vi "Grab Image and Find peoplel.vi"(8 "error in (no error)":errorcluster, 11 "ball tracking refs in":T2={"acquired image"=refnum, "threshold image"=refnum, "Video Handle out"=0, "Kinect Handle"=0, "Video and Depth config"={"Video Resolution"=enum."FREENECT_RESOLUTION_LOW", "Video Format"=enum."FREENECT_VIDEO_RGB", "Depth Format"=enum."FREENECT_DEPTH_11BIT", "Depth Resolution"=enum."FREENECT_RESOLUTION_MEDIUM"}}) -> (0 "error out":errorcluster, 1 "ball pixel position":T1, 2 "ball found?":bool, 3 "ball tracking refs out":T2={"acquired image"=refnum, "threshold image"=refnum, "Video Handle out"=0, "Kinect Handle"=0, "Video and Depth config"={"Video Resolution"=enum."FREENECT_RESOLUTION_LOW", "Video Format"=enum."FREENECT_VIDEO_RGB", "Depth Format"=enum."FREENECT_DEPTH_11BIT", "Depth Resolution"=enum."FREENECT_RESOLUTION_MEDIUM"}}, 4 "image resolution":cluster{"x":i32, "y":i32}={"x"=640, "y"=480})   [LabVIEW 2014]
doc: "This VI grabs an image from the camera, then estimates the locatation and distance of a green tennis ball in the image."
uses:
  Ball Tracking Image Refs.ctl
  <vilib>/vision/Image Controls.llb/IMAQ Image.ctl
  KinectProject/subVIs/Video Resolution Control.ctl
  KinectProject/subVIs/Video Format Control.ctl
  KinectProject/subVIs/Depth Format Control.ctl
  KinectProject/subVIs/Depth Resolution Control.ctl
  Ball Pixel Info.ctl
  Ball Tracking Globals.vi
  <vilib>/vision/NI_Vision_Development_Module.lvlib
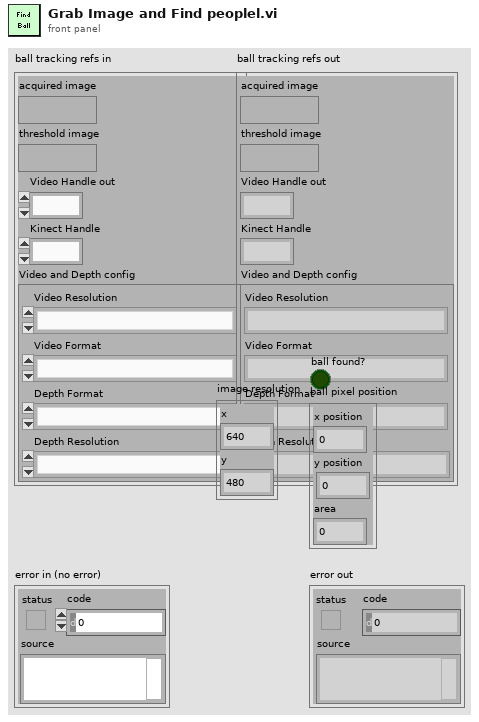
[diagram p1: front panel]
types:
  T1 = typedef "Ball Pixel Info.ctl" = cluster{"x position":dbl, "y position":dbl, "area":dbl}
  T2 = typedef "Ball Tracking Image Refs.ctl" = cluster{"acquired image":T3, "threshold image":T3, "Video Handle out":i64, "Kinect Handle":i64, "Video and Depth config":cluster{"Video Resolution":T4, "Video Format":T5, "Depth Format":T6, "Depth Resolution":T7}}
  T3 = typedef "IMAQ Image.ctl" = refnum<image>
  T4 = typedef "Video Resolution Control.ctl" = enum32{"FREENECT_RESOLUTION_LOW", "FREENECT_RESOLUTION_MEDIUM", "FREENECT_RESOLUTION_HIGH"}
  T5 = typedef "Video Format Control.ctl" = enum32{"FREENECT_VIDEO_RGB", "FREENECT_VIDEO_BAYER", "FREENECT_VIDEO_IR_8BIT", "FREENECT_VIDEO_IR_10BIT", "FREENECT_VIDEO_IR_10BIT_PACKED", "FREENECT_VIDEO_YUV_RGB", "FREENECT_VIDEO_YUV_RAW"}
  T6 = typedef "Depth Format Control.ctl" = enum32{"FREENECT_DEPTH_11BIT", "FREENECT_DEPTH_10BIT", "FREENECT_DEPTH_11BIT_PACKED", "FREENECT_DEPTH_10BIT_PACKED", "FREENECT_DEPTH_REGISTERED", "FREENECT_DEPTH_MM"}
  T7 = typedef "Depth Resolution Control.ctl" = enum16{"FREENECT_RESOLUTION_TINY", "FREENECT_RESOLUTION_LOW", "FREENECT_RESOLUTION_MEDIUM"}
  T8 = typedef "Particle Parameters" = i32
  T9 = cluster{"Video Resolution":T4, "Video Format":T5, "Depth Format":T6, "Depth Resolution":T7}
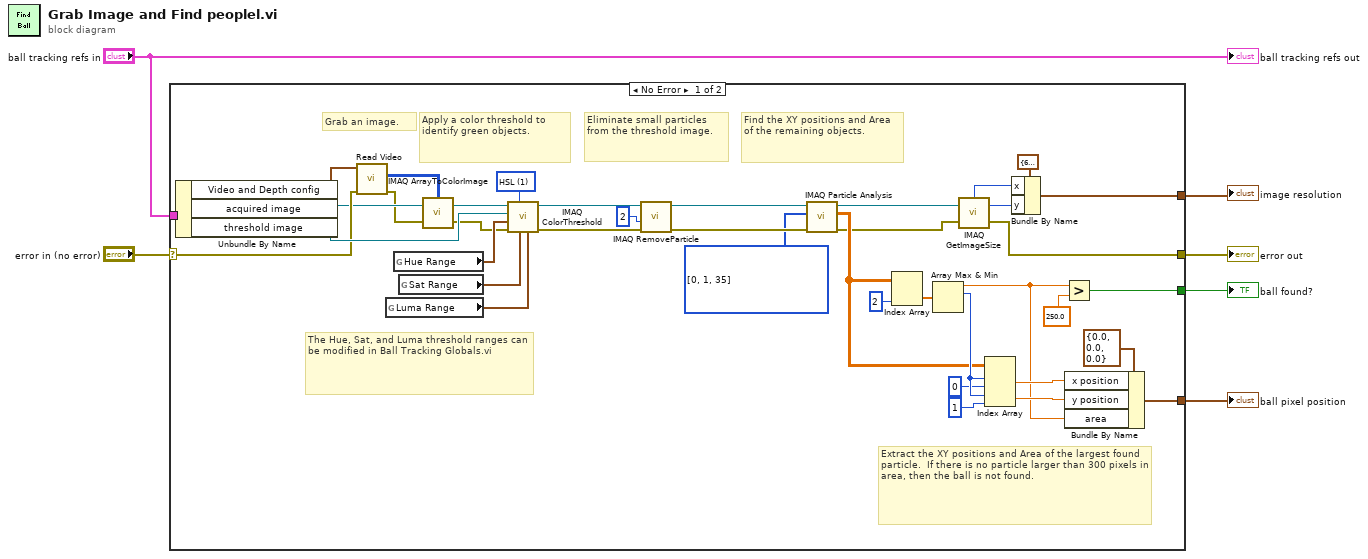
[diagram p0: block diagram]
diagram:
  n1 = case shown="No Error" "error in (no error)" {
    selector: "error in (no error)" -> [w13 w46]
    tunnel: "ball tracking refs in" -> [w45 _]
    tunnel: [w21 w46] -> w5
    tunnel: [w33 _] -> w3
    tunnel: [w25 _] -> w2
    tunnel: [w17 _] -> w1
    frame No Error {
      w37 = T8[] [0, 1, 35] items=["Center of Mass X", "Center of Mass Y", "First Pixel X", "First Pixel Y", "Bounding Rect Left", "Bounding Rect Top", "Bounding Rect Right", "Bounding Rect Bottom", "Max Feret Diameter Start X", "Max Feret Diameter Start Y", "Max Feret Diameter End X", "Max Feret Diameter End Y", "Max Horiz. Segment Length Left", "Max Horiz. Segment Length Right", "Max Horiz. Segment Length Row", "-", "Bounding Rect Width", "Bounding Rect Height", "Bounding Rect Diagonal", "Perimeter", "Convex Hull Perimeter", "Holes' Perimeter", "Max Feret Diameter", "Equivalent Ellipse Major Axis", "Equivalent Ellipse Minor Axis", "Equivalent Ellipse Minor Axis (Feret)", "Equivalent Rect Long Side", "Equivalent Rect Short Side", "Equivalent Rect Diagonal", "Equivalent Rect Short Side (Feret)", "Average Horiz. Segment Length", "Average Vert. Segment Length", "Hydraulic Radius", "Waddel Disk Diameter", "-", "Area", "Holes' Area", "Particle & Holes' Area", "Convex Hull Area", "Image Area", "-", "Number of Holes", "Number of Horiz. Segments", "Number of Vert. Segments", "-", "Orientation", "Max Feret Diameter Orientation", "-", "% Area/Image Area", "% Area/(Particle & Holes' Area)", "Ratio of Equivalent Ellipse Axes", "Ratio of Equivalent Rect Sides", "-", "Elongation Factor", "Compactness Factor", "Heywood Circularity Factor", "Type Factor", "-", "Sum X", "Sum Y", "Sum XX", "Sum XY", "Sum YY", "Sum XXX", "Sum XXY", "Sum XYY", "Sum YYY", "-", "Moment of Inertia XX", "Moment of Inertia XY", "Moment of Inertia YY", "Moment of Inertia XXX", "Moment of Inertia XXY", "Moment of Inertia XYY", "Moment of Inertia YYY", "Norm. Moment of Inertia XX", "Norm. Moment of Inertia XY", "Norm. Moment of Inertia YY", "Norm. Moment of Inertia XXX", "Norm. Moment of Inertia XXY", "Norm. Moment of Inertia XYY", "Norm. Moment of Inertia YYY", "Hu Moment 1", "Hu Moment 2", "Hu Moment 3", "Hu Moment 4", "Hu Moment 5", "Hu Moment 6", "Hu Moment 7"] ("Pixel Measurements")
      w43 = u16 1 items=["RGB", "HSL", "HSV", "HSI"] ("Color Mode")
      # "The Hue, Sat, and Luma threshold ranges can be modified in Ball Tracking Globals.vi"
      # "Extract the XY positions and Area of the largest found particle.  If there is no particle larger than 300 pixels in area, then the ball is not found."
      # "Find the XY positions and Area of the remaining objects."
      # "Eliminate small particles from the threshold image."
      # "Apply a color threshold to identify green objects."
      # "Grab an image."
      n2 = Unbundle By Name(w45) -> ("Video and Depth config"=w12:T9, "acquired image"=w11:T3, "threshold image"=w44:T3)
      n3 = call "Read Video.vi"("error in (no error)"=w13, "input cluster"=w12) -> ("error out"=w9:errorcluster, "video"=w7:u32[][])  [unwired: 6 in, 2 out]
      n4 = global read "Ball Tracking Globals.vi" "Luma Range"() -> (w14:cluster{"Lower value":i32, "Upper value":i32})
      n5 = global read "Ball Tracking Globals.vi" "Hue Range"() -> (w16:cluster{"Lower value":i32, "Upper value":i32})
      n6 = global read "Ball Tracking Globals.vi" "Sat Range"() -> (w15:cluster{"Lower value":i32, "Upper value":i32})
      n7 = call "IMAQ ArrayToColorImage"("Image Pixels (U32)"=w7, "Image"=w11, "error in (no error)"=w9) -> ("Image Out"=w10:T3, "error out"=w8:errorcluster)  [unwired: 2 in]
      n8 = call "IMAQ ColorThreshold"("Blue or Luma or Val or Inten Range"=w14, "Green or Sat Range"=w15, "Color Mode"=w43, "error in (no error)"=w8, "Red or Hue Range"=w16, "Image Dst"=w44, "Image Src"=w10) -> ("error out"=w40:errorcluster, "Image Dst Out"=w41:T3)  [unwired: 3 in]
      n9 = call "IMAQ RemoveParticle"("error in (no error)"=w40, "Number of Erosion"=2, "Image Src"=w41) -> ("error out"=w38:errorcluster, "Image Dst Out"=w39:T3)  [unwired: 7 in]
      n10 = call "IMAQ Particle Analysis"("error in (no error)"=w38, "Pixel Measurements"=w37, "Image"=w39) -> ("error out"=w22:errorcluster, "Particle Measurements (Pixels)"=w29:dbl[][], "Image Out (duplicate)"=w23:T3)  [unwired: 3 in, 3 out]
      n11 = Index Array(array=w29, index (col)=2 ("disabled index (col)")) -> (element=w36:dbl[])  [unwired: 1 in]
      n12 = Array Max & Min(array=w36) -> (max value=w24:dbl, max index (indices)=w32:i32)  [unwired: 2 out]
      n13 = call "IMAQ GetImageSize"("Image"=w23, "error in (no error)"=w22) -> ("Y Resolution"=w18:i32, "X Resolution"=w19:i32, "error out"=w21:errorcluster)  [unwired: 2 in]
      n14 = Index Array(array=w29, index (row) #1=w32, index (col) #1=0 ("index (col)"), index (row) #2=w32, index (col) #2=1 ("index (col)")) -> (element #1=w27:dbl, element #2=w26:dbl)
      n15 = Bundle By Name(cluster=cluster{"x":i32, "y":i32} {"x"=640, "y"=480} ("image resolution"), "x"=w19, "y"=w18) -> (w17:cluster{"x":i32, "y":i32})
      n16 = Greater?(x=w24, y=250.0) -> (0:w33:bool)
      n17 = Bundle By Name(cluster=T1 {"x position"=0.0, "y position"=0.0, "area"=0.0} ("pixel info"), "x position"=w27, "y position"=w26, "area"=w24) -> (w25:T1)
    }
    frame Error {
    }
  }
  "error out" <- w5
  "ball found?" <- w3
  "ball pixel position" <- w2
  "image resolution" <- w1
  "ball tracking refs out" <- "ball tracking refs in"
